vi "ultrasonic.vi"() -> ()   [LabVIEW 2024]
uses:
  <vilib>/Instr/_visa.llb/VISA Configure Serial Port (Instr).vi
panel:
  out "buzzer":bool
  out "distance":dbl(graph)
  out "green LED":bool caption="Red LED"
  out "BlueLED":bool
  out "red LED":bool
  out "Humidity":dbl(graph)
  out "Humidity":dbl(slide) scale=0.0..100.0
  out "Distance":dbl(knob) scale=0.0..400.0
  in  "stop":bool
  in  "parity (0:none)":enum16{"None", "Odd", "Even", "Mark", "Space"}(ring)
  in  "data bits (8)":u16=8 min=5 max=8 step=1
  in  "baud rate (250000)":u32=9600
  in  "VISA resource name":refnum<visa-resource-name>
  out "Boolean 3":bool
  out "Boolean":bool
  out "Temperature":dbl(slide) scale=0.0..100.0
  out "temperature":dbl(graph)
  out "Exaust Fan":bool
  out "boolean 3":bool
  out "Boolean 8":bool
  out "Boolean 7":bool
  out "Boolean 6":bool
  out "Boolean 5":bool
  out "Boolean 4":bool
  out "Boolean 2":bool
  out "Exaust valve":bool
  out "PUMP":bool
  out "gas":dbl(graph)
  out "Gas Values":dbl(slide) scale=0.0..1000.0
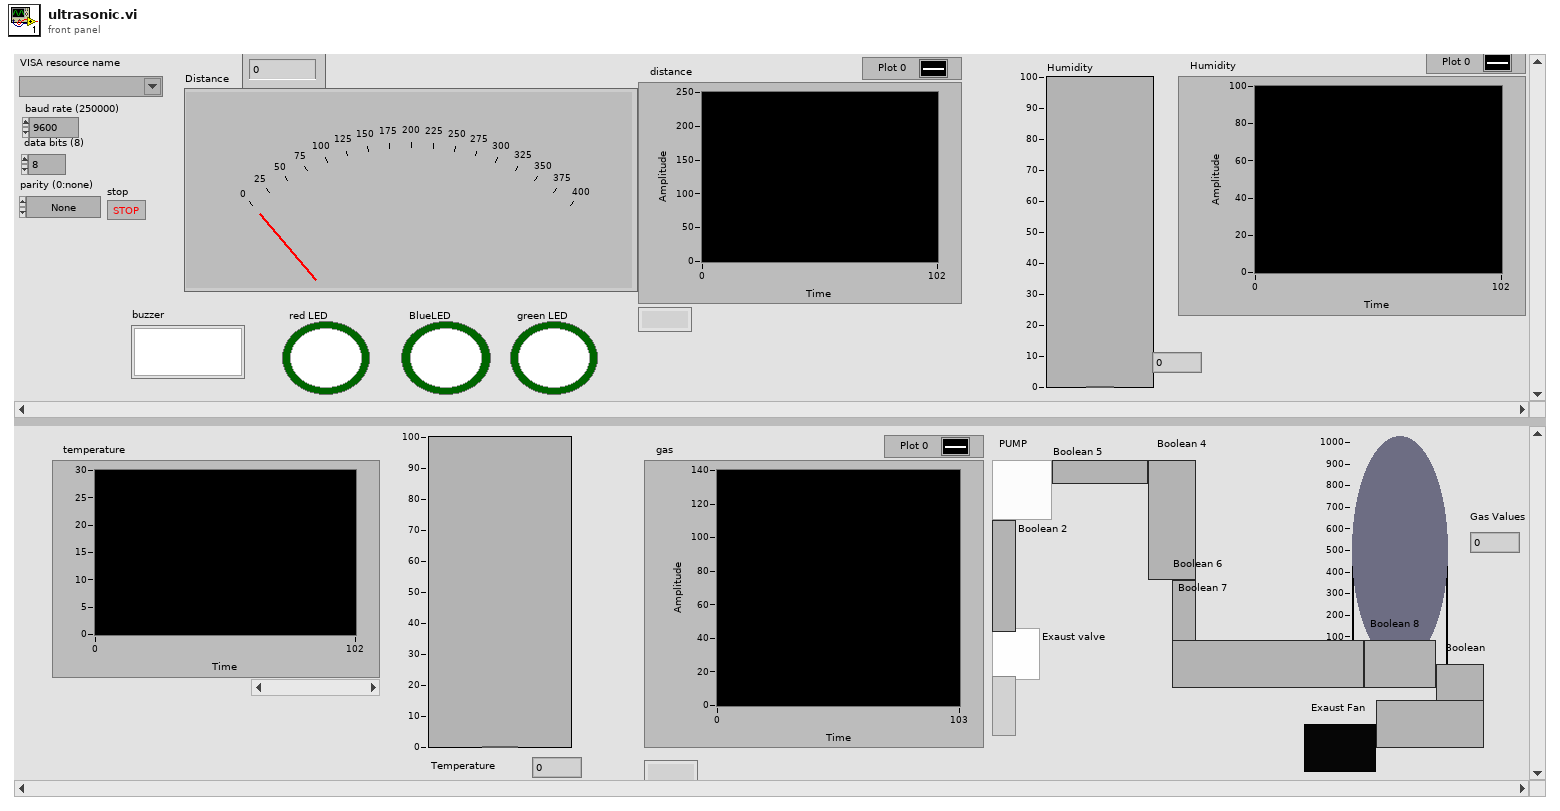
[diagram p1: front panel]
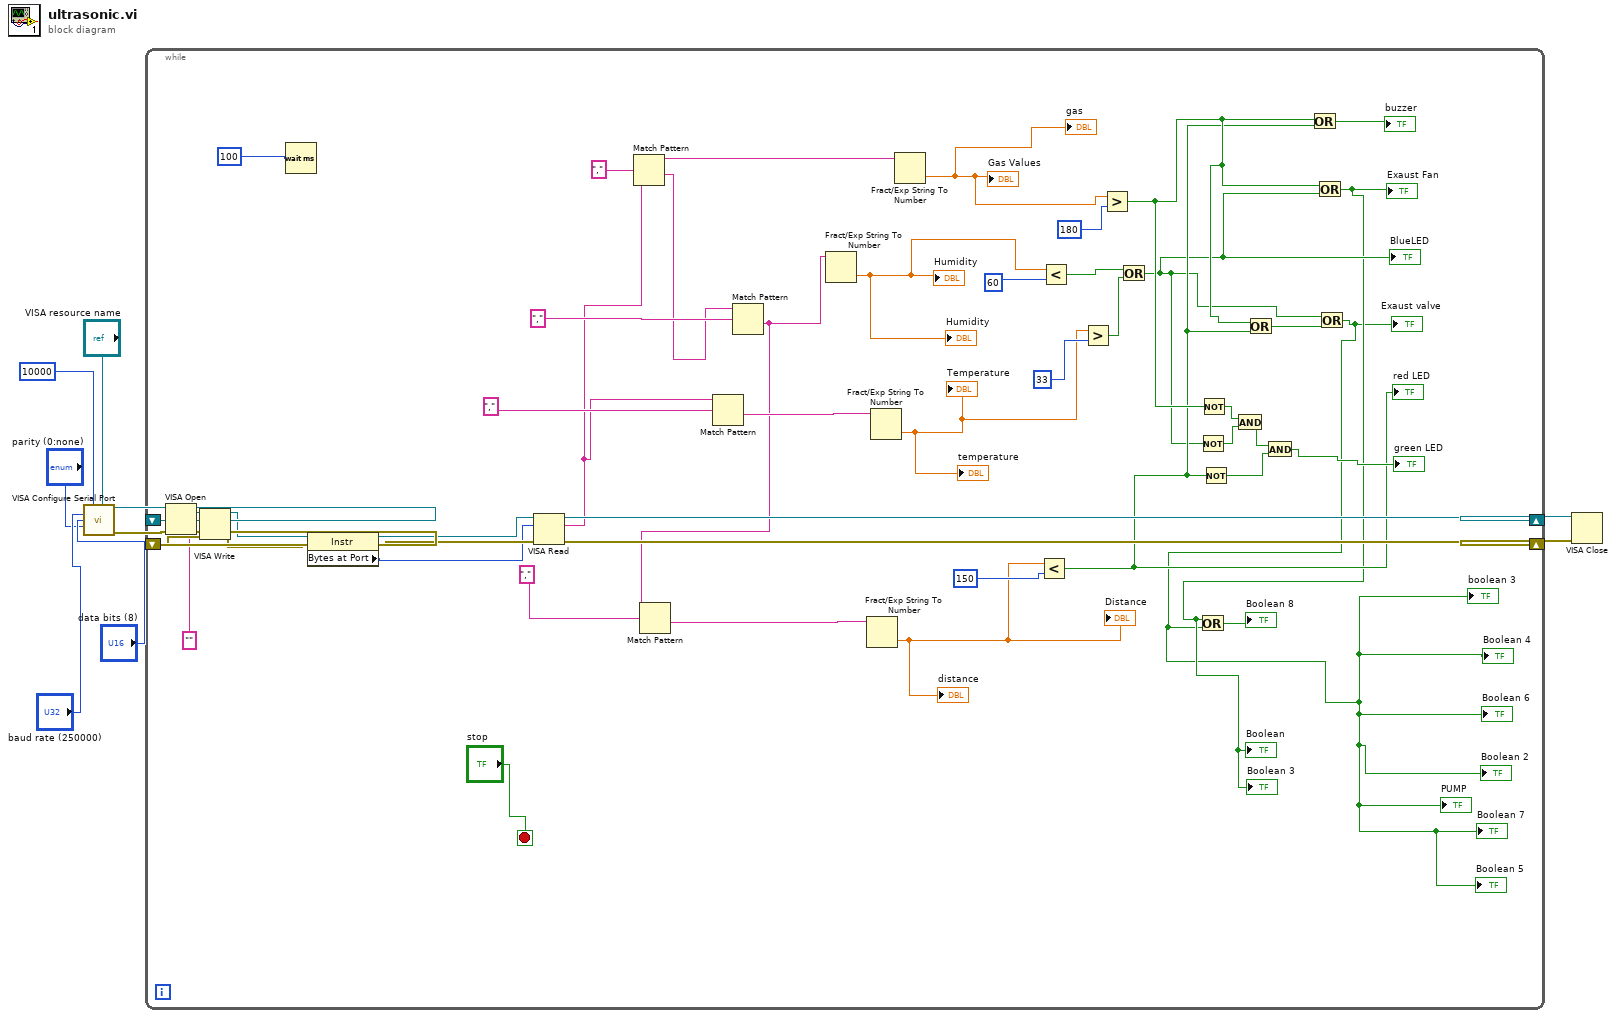
[diagram p0: block diagram]
diagram:
  n1 = call-poly "VISA Configure Serial Port"("VISA resource name"="VISA resource name", "timeout (10sec)"=u32 10000, "baud rate (9600)"="baud rate (250000)", "data bits (8)"="data bits (8)", "parity (0:none)"="parity (0:none)") -> ("VISA resource name out"=w11:refnum<visa-resource-name>, "error out"=w10:errorcluster)  [unwired: 9 in]
  n2 = VISA Open(error in (no error)=w10, VISA resource name=w11) -> (VISA resource name=w9:refnum<visa-resource-name>, error out=w8:errorcluster)  [unwired: 3 in]
  n3 = while {
    shift-right: [w55] -> w7
    shift-left: w9 -> [w54]
    shift-right: [w37] -> w6
    shift-left: w8 -> [w53]
    stop <- "stop" stop-if-true
    n4 = VISA Write(VISA resource name=w54, write buffer="", error in (no error)=w53) -> (VISA resource name out=w52:refnum<visa-resource-name>, error out=w51:errorcluster)  [unwired: 1 out]
    n5 = Wait (ms)(milliseconds to wait=u32 100) -> ()  [unwired: 1 out]
    n6 = property class="Instr"(reference=w52, error in=w51) -> (reference out=w50:refnum<visa-resource-name>, error out=w49:errorcluster, "Bytes at Port"=w48:u32)
    n7 = VISA Read(VISA resource name=w50, byte count=w48, error in (no error)=w49) -> (VISA resource name out=w55:refnum<visa-resource-name>, read buffer=w39:string, error out=w37:errorcluster)  [unwired: 1 out]
    n8 = Match Pattern(string=w39, regular expression=",") -> (before substring=w40:string, after substring=w38:string)  [unwired: 1 in, 2 out]
    n9 = Match Pattern(string=w39, regular expression=",") -> (after substring=w41:string)  [unwired: 1 in, 3 out]
    n10 = Match Pattern(string=w38, regular expression=",") -> (after substring=w36:string)  [unwired: 1 in, 3 out]
    n11 = Match Pattern(string=w36, regular expression=",") -> (after substring=w46:string)  [unwired: 1 in, 3 out]
    n12 = Fract/Exp String To Number(string=w36) -> (number=w13:dbl)  [unwired: 3 in, 1 out]
    "Humidity" <- w13
    "Humidity" <- w13
    n13 = Fract/Exp String To Number(string=w46) -> (number=w14:dbl)  [unwired: 3 in, 1 out]
    "Distance" <- w14
    "distance" <- w14
    n14 = Fract/Exp String To Number(string=w41) -> (number=w15:dbl)  [unwired: 3 in, 1 out]
    "Temperature" <- w15
    "temperature" <- w15
    n15 = Fract/Exp String To Number(string=w40) -> (number=w12:dbl)  [unwired: 3 in, 1 out]
    "Gas Values" <- w12
    "gas" <- w12
    n16 = Less?(x=w14, y=150) -> (x < y?=w19:bool)
    "red LED" <- w19
    n17 = Less?(x=w13, y=60) -> (x < y?=w26:bool)
    n18 = Greater?(x=w15, y=33) -> (0:w27:bool)
    n19 = Greater?(x=w12, y=180) -> (0:w21:bool)
    n20 = Or(x=w26, y=w27) -> (x .or. y?=w18:bool)
    "BlueLED" <- w18
    n21 = Not(x=w18) -> (.not. x?=w24:bool)
    n22 = Not(x=w21) -> (.not. x?=w25:bool)
    n23 = Not(x=w19) -> (.not. x?=w23:bool)
    n24 = And(x=w25, y=w24) -> (x .and. y?=w22:bool)
    n25 = Or(x=w21, y=w19) -> (x .or. y?=w28:bool)
    n26 = And(x=w22, y=w23) -> (x .and. y?=→"green LED":bool)
    n27 = Or(x=w21, y=w19) -> (x .or. y?=→"buzzer":bool)
    n28 = Or(x=w21, y=w18) -> (x .or. y?=w17:bool)
    "Exaust Fan" <- w17
    "Boolean" <- w17
    "Boolean 3" <- w17
    n29 = Or(x=w18, y=w28) -> (x .or. y?=w16:bool)
    "PUMP" <- w16
    "Exaust valve" <- w16
    "Boolean 2" <- w16
    "Boolean 4" <- w16
    "Boolean 5" <- w16
    "Boolean 6" <- w16
    "Boolean 7" <- w16
    "boolean 3" <- w16
    n30 = Or(x=w17, y=w16) -> (x .or. y?=→"Boolean 8":bool)
  }
  n31 = VISA Close(VISA resource name=w7, error in (no error)=w6) -> ()  [unwired: 1 out]
